vi "SENS_CORR_PREF_ECAL_ORI_STAT.vi"(0 "VISA IN":refnum<visa-resource-name>, 1 "On/Off":bool, 5 "error in":errorcluster, 7 "Channel":i32) -> (14 "VISA Out":refnum<visa-resource-name>, 19 "error out":errorcluster)   [LabVIEW 2018, in "PNA-X.lvlib"]
doc: "SENSe<cnum>:CORRection:COLLect:ISOLation:ECAL:[:STATe] <bool> \n(Read-Write) Specifies whether or not the isolation state of the ECal module will be measured as part \nof an unguided ECal calibration. \nAn unguided calibration is performed using the SENS:CORR:COLL:METH and \nSENS:CORR:COLL:ACQ commands. \nNote: The inherent isolation of the PNA is better than that attained with this command. ONLY use \nthis command when using an external test set, and ONLY using a 8509x ECal module. \nParameters \n<cnum> Any existing channel number. If unspecified, value is set to 1 \n<bool> ON (or 1) - isolation is measured during the unguided ECal calibration. \nOFF (or 0) isolation is NOT measured during the unguided ECal calibration. \nExamples SENS1:CORR:COLL:ISOL:ECAL ON \nsense2:correction:collect:isolation:ecal:state 0 \nQuery Syntax SENSe:CORRection:COLLect:ISOLation:ECAL:STATe? \nReturn Type Boolean (1 = ON, 0 = OFF) \nDefault OFF \n1629"
uses:
  PNA-X.lvlib
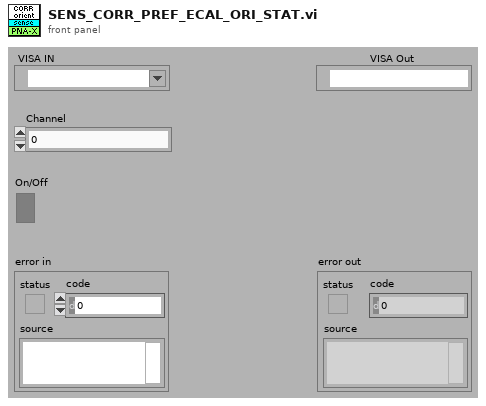
[diagram p1: front panel]
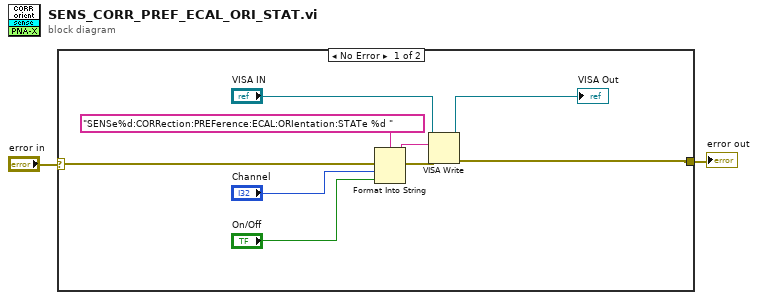
[diagram p0: block diagram]
diagram:
  n1 = case shown="No Error" "error in" {
    selector: "error in" -> [w11 w12]
    tunnel: [w6 w12] -> w1
    frame No Error {
      n2 = Format Into String(format string="SENSe%d:CORRection:PREFerence:ECAL:ORIentation:STATe %d " ("Cmdline"), error in=w11, "Channel", "On/Off") -> (resulting string=w9:string, error out=w10:errorcluster)  [unwired: 1 in]
      n3 = VISA Write(VISA resource name="VISA IN", write buffer=w9, error in (no error)=w10) -> (VISA resource name out=→"VISA Out":refnum<visa-resource-name>, error out=w6:errorcluster)  [unwired: 1 out]
    }
    frame Error {
    }
  }
  "error out" <- w1
